vi "DEMO-Read Mem.vi"() -> ()   [LabVIEW 2016]
uses:
  <userlib>/LV-JLinkARM/JLinkARM.lvlib
panel:
  in  "Device":string(combo)="STM32F407ZG"
  out "buff":u8[](array[numeric]) format="%02x"
  in  "size":u32
  in  "memaddr":u32=536870912 format="%08x"
  out "function return":i32
  out "error out":errorcluster
  in  "error in (no error)":errorcluster caption="错误输入（无错误）"
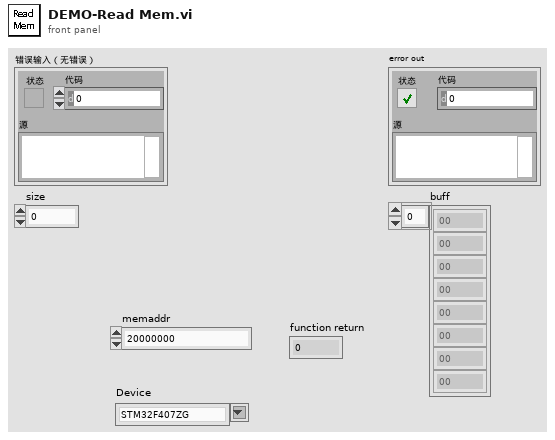
[diagram p1: front panel]
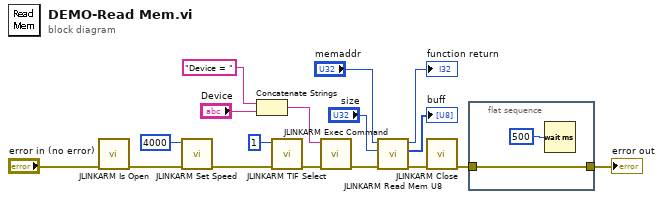
[diagram p0: block diagram]
diagram:
  n1 = call <userlib>:"JLINKARM Is Open.vi"("error in (no error)"="error in (no error)") -> ("error out"=w7:errorcluster)  [unwired: 9 in, 1 out]
  n2 = call <userlib>:"JLINKARM Set Speed.vi"("error in (no error)"=w7, "jlink_speed"=u32 4000) -> ("error out"=w6:errorcluster)  [unwired: 8 in, 1 out]
  n3 = Concatenate Strings("Device = " ("pbCommand"), "Device") -> (w1:string)
  n4 = call <userlib>:"JLINKARM TIF Select.vi"("error in (no error)"=w6, "is_swd_intf"=u32 1) -> ("error out"=w12:errorcluster)  [unwired: 8 in, 1 out]
  n5 = call <userlib>:"JLINKARM Exec Command.vi"("error in (no error)"=w12, "pbCommand"=w1) -> ("error out"=w15:errorcluster)  [unwired: 7 in, 2 out]
  n6 = call <userlib>:"JLINKARM Read Mem U8.vi"("error in (no error)"=w15, "size"="size", "memaddr"="memaddr") -> ("error out"=w14:errorcluster, "buff"=→"buff":u8[], "function return"=→"function return":i32)  [unwired: 6 in]
  n7 = call <userlib>:"JLINKARM Close.vi"("error in (no error)"=w14) -> ("error out"=w13:errorcluster)  [unwired: 9 in, 1 out]
  n8 = flat-sequence {
    tunnel: [w18] -> w16
    tunnel: w13 -> [w18]
    frame #0 {
      n9 = Wait (ms)(milliseconds to wait=u32 500 ("等待时间（毫秒）")) -> ()  [unwired: 1 out]
    }
  }
  "error out" <- w16
